vi "GVZwangsMPV.vi"() -> ()   [LabVIEW 2010]
panel:
  out "ZwangsMPV?":bool
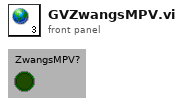
[diagram p1: front panel]
diagram:
